vi "oa_Even Angle Signal Delay Processing.vi"(7 "reset? (T)":bool=TRUE, 9 "number of points":i32, 11 "even angle signal in":cluster{"r0":dbl, "dr":dbl, "Y":dbl[]}={"r0"=0.0, "dr"=1.0, "Y"=[]} {"r0" format="%.2p"; "dr" format="%.2p"; "Y" format="%.2f"}) -> (3 "buffered even angle signal":cluster{"r0":dbl, "dr":dbl, "Y":dbl[]}={"r0"=0.0, "dr"=1.0, "Y"=[]} {"r0" format="%.2p"; "dr" format="%.2p"; "Y" format="%.2f"})   [LabVIEW 2017, in "SoundVib_OAUtility.lvlib"]
uses:
  <vilib>/addons/Sound and Vibration/Order Analysis/Utility/SoundVib_OAUtility.lvlib
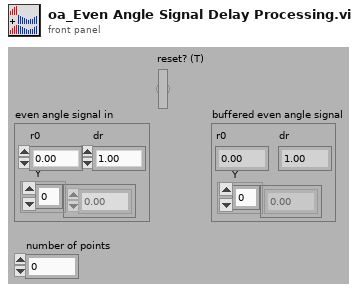
[diagram p1: front panel]
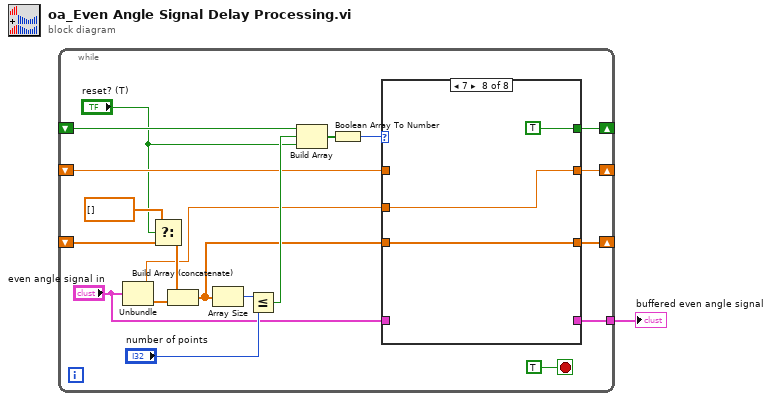
[diagram p0: block diagram]
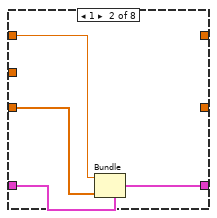
[diagram p3: hidden frame]
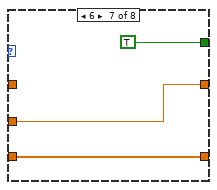
[diagram p8: hidden frame]
diagram:
  n1 = while {
    shift-right: [w14] -> _
    shift-left: _ -> [w3]
    shift-right: [w4] -> _
    shift-left: _ -> [w7]
    shift-right: [w6] -> _
    shift-left: _ -> [w11]
    tunnel: [w12] -> w1
    stop <- TRUE stop-if-true
    n2 = Unbundle("even angle signal in") -> ("r0"=w5:dbl, "Y"=w18:dbl[])  [unwired: 1 out]
    n3 = Select(t=dbl[] [] ("Y"), s="reset? (T)", f=w11) -> (s? t:f=w9:dbl[])
    n4 = Build Array (concatenate)(w9, w18) -> (w8:dbl[])
    n5 = Array Size(array=w8) -> (size(s)=w20:i32)
    n6 = Less Or Equal?(x=w20, y="number of points") -> (x <= y?=w17:bool)
    n7 = Build Array(w3, w17, "reset? (T)") -> (w16:bool[])
    n8 = Boolean Array To Number(Boolean array=w16) -> (number=w15:u32)
    n9 = case shown="7" w15 {
      tunnel: [_ _ _ _ _ _ TRUE TRUE] -> w14
      tunnel: "even angle signal in" -> [w22 w25 w27 _ w30 w31 _ _]
      tunnel: [w22 w26 w27 _ w30 w31 _ _] -> w12
      tunnel: w8 -> [_ w24 _ w29 _ _ w33 w36]
      tunnel: w7 -> [_ w23 _ w28 _ _ _ _]
      tunnel: [_ _ _ w29 _ _ w33 w36] -> w6
      tunnel: w5 -> [_ _ _ _ _ _ w34 w37]
      tunnel: [_ _ _ w28 _ _ w34 w37] -> w4
      frame 0, Default {
      }
      frame 1 {
        n10 = Bundle(cluster=w25, "r0"=w23, "Y"=w24) -> (w26:cluster{"r0":dbl, "dr":dbl, "Y":dbl[]})  [unwired: 1 in]
      }
      frame 2 {
      }
      frame 3 {
      }
      frame 4 {
      }
      frame 5 {
      }
      frame 6 {
      }
      frame 7 {
      }
    }
  }
  "buffered even angle signal" <- w1
